vi "4 -1 - Save transition data rally seperated.vi"() -> ()   [LabVIEW 2013]
uses:
  <vilib>/Utility/file.llb/Read From Spreadsheet File (DBL).vi
panel:
  in  "Player position segment data":path
  in  "Startend":path
  in  "XY and frame data":path
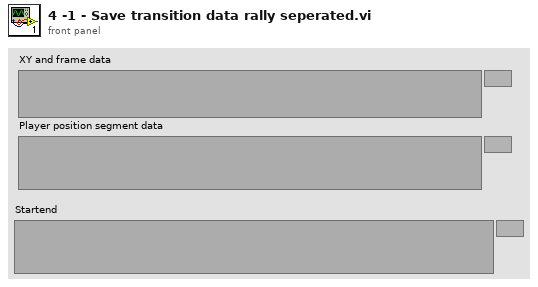
[diagram p1: front panel]
types:
  T1 = enum16{"open", "replace", "create", "open or create", "replace or create", "replace or create with confirmation"}
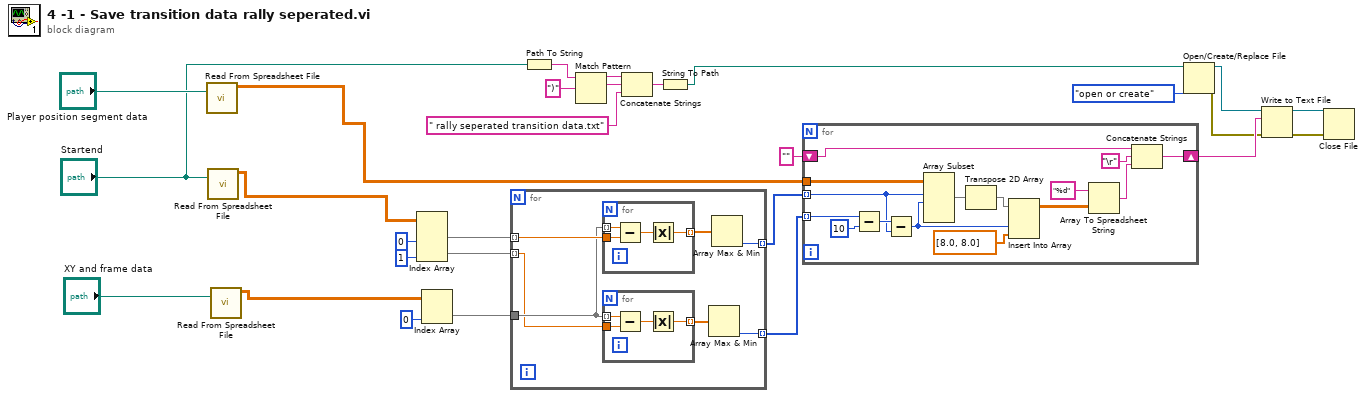
[diagram p0: block diagram]
diagram:
  n1 = call-poly <vilib>:"Read From Spreadsheet File.vi"("file path (dialog if empty)"="Player position segment data") -> ("all rows"=w11:dbl[][])  [unwired: 6 in, 4 out]
  n2 = call-poly <vilib>:"Read From Spreadsheet File.vi"("file path (dialog if empty)"="Startend") -> ("all rows"=w10:dbl[][])  [unwired: 6 in, 4 out]
  n3 = call-poly <vilib>:"Read From Spreadsheet File.vi"("file path (dialog if empty)"="XY and frame data") -> ("all rows"=w9:dbl[][])  [unwired: 6 in, 4 out]
  n4 = Index Array(array=w10, index (col) #1=0 ("disabled index (col)"), index (col) #2=1 ("index (col)")) -> (element #1=w26:dbl[], element #2=w25:dbl[])  [unwired: 2 in]
  n5 = Index Array(array=w9, index (col)=0 ("disabled index (col)")) -> (element=w23:dbl[])  [unwired: 1 in]
  n6 = for {
    tunnel: w26 -> [w35] mode=indexing
    tunnel: w25 -> [w30] mode=indexing
    tunnel: w23 -> [w31]
    tunnel: [w33] -> w22 mode=indexing
    tunnel: [w32] -> w21 mode=indexing
    n7 = for {
      tunnel: w35 -> [w42]
      tunnel: w31 -> [w43] mode=indexing
      tunnel: [w40] -> w34 mode=indexing
      n8 = Subtract(x=w43, y=w42) -> (x-y=w41:dbl)
      n9 = Absolute Value(x=w41) -> (abs(x)=w40:dbl)
    }
    n10 = for {
      tunnel: w30 -> [w38]
      tunnel: w31 -> [w39] mode=indexing
      tunnel: [w36] -> w29 mode=indexing
      n11 = Subtract(x=w39, y=w38) -> (x-y=w37:dbl)
      n12 = Absolute Value(x=w37) -> (abs(x)=w36:dbl)
    }
    n13 = Array Max & Min(array=w29) -> (min index (indices)=w32:i32)  [unwired: 3 out]
    n14 = Array Max & Min(array=w34) -> (min index (indices)=w33:i32)  [unwired: 3 out]
  }
  n15 = Path To String(path="Startend") -> (string=w7:string)
  n16 = Match Pattern(string=w7, regular expression=")") -> (before substring=w5:string, match substring=w4:string)  [unwired: 1 in, 2 out]
  n17 = Concatenate Strings(w5, w4, " rally seperated transition data.txt" ("regular expression")) -> (w3:string)
  n18 = String To Path(string=w3) -> (path=w1:path)
  n19 = for {
    tunnel: w22 -> [w54] mode=indexing
    tunnel: w21 -> [w55] mode=indexing
    tunnel: w11 -> [w56]
    shift-right: [w48] -> w17
    shift-left: "" ("spreadsheet string") -> [w50]
    n20 = Subtract(x=w55, y=10) -> (x-y=w58:i32)
    n21 = Subtract(x=w58, y=w54) -> (x-y=w44:i32)
    n22 = Array Subset(array=w56, index (row)=w54, length (row)=w44) -> (w52:dbl[][])  [unwired: 2 in]
    n23 = Transpose 2D Array(2D array=w52) -> (transposed array=w47:dbl[][])
    n24 = Insert Into Array(array=w47, index (col)=w44, new element=dbl[] [8.0, 8.0] ("new element/subarray")) -> (w45:dbl[][])  [unwired: 1 in]
    n25 = Array To Spreadsheet String(array=w45, 3:"%d" ("format string")) -> (spreadsheet string=w49:string)  [unwired: 1 in]
    n26 = Concatenate Strings(w50, "\r", w49) -> (w48:string)
  }
  n27 = Open/Create/Replace File(file path (use dialog)=w1, operation (0:open)=T1."open or create") -> (refnum out=w19:refnum<file>, error out=w15:errorcluster)  [unwired: 4 in, 1 out]
  n28 = Write to Text File(file (use dialog)=w19, text=w17, error in=w15) -> (refnum out=w18:refnum<file>, error out=w16:errorcluster)  [unwired: 1 in, 1 out]
  n29 = Close File(refnum=w18, error in=w16) -> ()  [unwired: 2 out]
